vi "Insert Edge Point (by index).vi"(0 "FSM.Graph In":refnum<class "FSM.Graph.lvclass">, 5 "Location":cluster{"x":i16, "y":i16}, 7 "edgeIndex":i32, 9 "Even space":bool=TRUE) -> (4 "FSM.Graph Out":refnum<class "FSM.Graph.lvclass">)   [LabVIEW 2020, in "FSM.Graph.lvclass"]
uses:
  FSM.Graph.lvclass
  FSM.Graph.lvclass/FSM.Graph.ctl
  FSM.Edge/FSM.Edge.lvclass
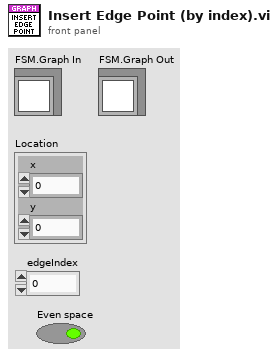
[diagram p1: front panel]
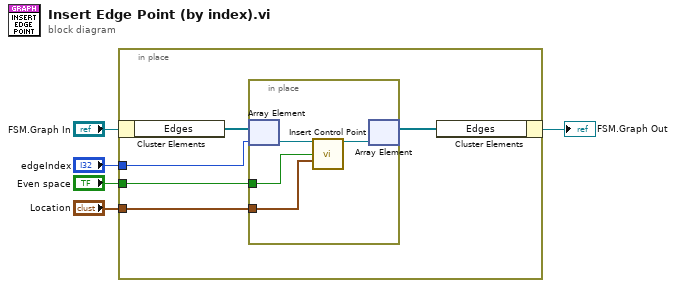
[diagram p0: block diagram]
diagram:
  n1 = in-place {
    in-place-border: "edgeIndex" -> [w10]
    in-place-border: "Location" -> [w9]
    in-place-border: "Even space" -> [w6]
    n2 = in-place-cluster #1("FSM.Graph In") -> ("Edges"=w7:refnum<class "FSM.Edge.lvclass">[])
    n3 = in-place {
      in-place-border: w9 -> [w12]
      in-place-border: w6 -> [w11]
      n4 = in-place-array #2(w7, w10) -> (w14:refnum<class "FSM.Edge.lvclass">)
      n5 = call "Insert Control Point.vi"("FSM.Edge In"=w14, "Even space"=w11, "location"=w12) -> ("FSM.Edge Out"=w13:refnum<class "FSM.Edge.lvclass">)  [unwired: 12 in]
      n6 = in-place-array #2(w13) -> (w8:refnum<class "FSM.Edge.lvclass">[])  [unwired: 1 out]
    }
    n7 = in-place-cluster #1("Edges"=w8) -> (→"FSM.Graph Out":refnum<class "FSM.Graph.lvclass">)
  }
